vi "Write Double.vi"(8 "error in (no error)":errorcluster, 9 "Data":dbl, 10 "Channel Index":i32, 11 "CIFChannelMng in":refnum<class "CIFChannelMng.lvclass">) -> (0 "error out":errorcluster, 1 "timed out?":bool, 3 "CIFChannelMng out":refnum<class "CIFChannelMng.lvclass">)   [LabVIEW 2021, in "CIFChannelMng.lvclass"]
uses:
  CIFChannelMng.lvclass
  CIFChannelMng.lvclass/CIFChannelMng.ctl
  CIFChannels/CIFChannels.lvclass
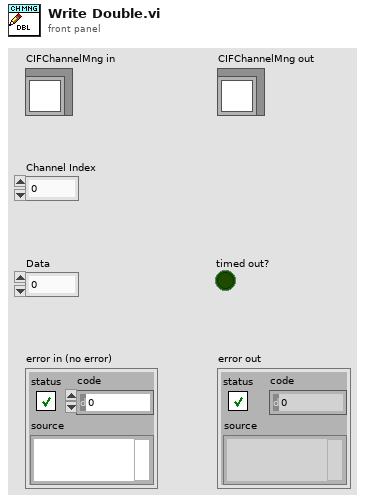
[diagram p1: front panel]
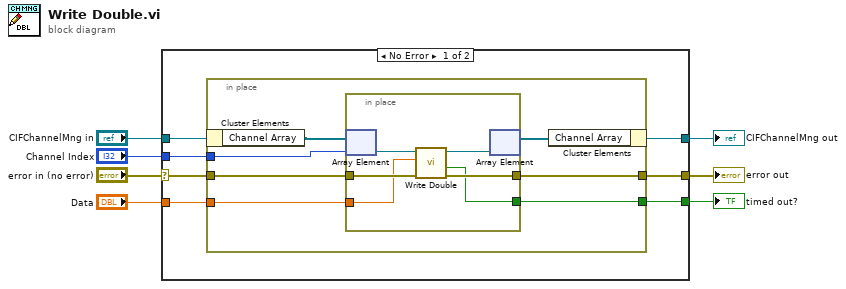
[diagram p0: block diagram]
diagram:
  n1 = case shown="No Error" "error in (no error)" {
    selector: "error in (no error)" -> [w12 w29]
    tunnel: [w11 w29] -> w6
    tunnel: [w13 w28] -> w4
    tunnel: "CIFChannelMng in" -> [w14 w28]
    tunnel: "Data" -> [w10 _]
    tunnel: [w9 _] -> w2
    tunnel: "Channel Index" -> [w8 _]
    frame No Error {
      n2 = in-place {
        in-place-border: w12 -> [w21]
        in-place-border: [w15] -> w11
        in-place-border: w10 -> [w20]
        in-place-border: [w19] -> w9
        in-place-border: w8 -> [w16]
        n3 = in-place-cluster #1(w14) -> ("Channel Array"=w18:refnum<class "CIFChannels.lvclass">[])
        n4 = in-place {
          in-place-border: w21 -> [w27]
          in-place-border: [w26] -> w15
          in-place-border: [w25] -> w19
          in-place-border: w20 -> [w24]
          n5 = in-place-array #2(w18, w16) -> (w23:refnum<class "CIFChannels.lvclass">)
          n6 = call-dynamic "Write Double.vi"("error in (no error)"=w27, "Data"=w24, "CIFChannels in"=w23) -> ("error out"=w26:errorcluster, "timed out?"=w25:bool, "CIFChannels out"=w22:refnum<class "CIFChannels.lvclass">)  [unwired: 6 in]
          n7 = in-place-array #2(w22) -> (w17:refnum<class "CIFChannels.lvclass">[])  [unwired: 1 out]
        }
        n8 = in-place-cluster #1("Channel Array"=w17) -> (w13:refnum<class "CIFChannelMng.lvclass">)
      }
    }
    frame Error {
    }
  }
  "error out" <- w6
  "CIFChannelMng out" <- w4
  "timed out?" <- w2
